vi "PythagFindB.vi"(1 "Side B":dbl, 2 "Side H":dbl) -> (0 "Side B":dbl)   [LabVIEW 2016]
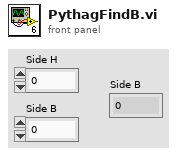
[diagram p1: front panel]
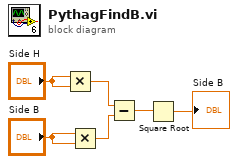
[diagram p0: block diagram]
diagram:
  n1 = Multiply(x="Side H", y="Side H") -> (x*y=w4:dbl)
  n2 = Multiply(x="Side B", y="Side B") -> (x*y=w3:dbl)
  n3 = Subtract(x=w4, y=w3) -> (x-y=w2:dbl)
  n4 = Square Root(x=w2) -> (sqrt(x)=→"Side B":dbl)
